vi "Test_Observe_NoPublication_Timeout.vi"(8 "error in (no error)":errorcluster, 11 "TestObservation In":refnum<class "TestPubSubRouting.lvclass">) -> (0 "error out":errorcluster, 3 "TestObservation Out":refnum<class "TestPubSubRouting.lvclass">)   [LabVIEW 2017, in "TestPubSubRouting.lvlib" / "TestPubSubRouting.lvclass"]
uses:
  TestPubSubRouting.lvclass
  gpm_packages/@cs/mva-core/Source/Mediator/Mediator/Mediator.lvclass
  <vilib>/ActorFramework/Actor/Actor.lvclass
  ObservingViewable/ObservingViewable.lvclass
  <vilib>/ActorFramework/Stop Msg/Stop Msg.lvclass
  ObservingViewModel/ObservingViewModel.lvclass
  ObservingModel/ObservingModel.lvclass
  41be6b66-6851-409e-b7f3-4ca1eaa927d9.vi
  C:/Program Files (x86)/National Instruments/LabVIEW 2017/vi.lib/ActorFramework/Actor/Actor.lvclass
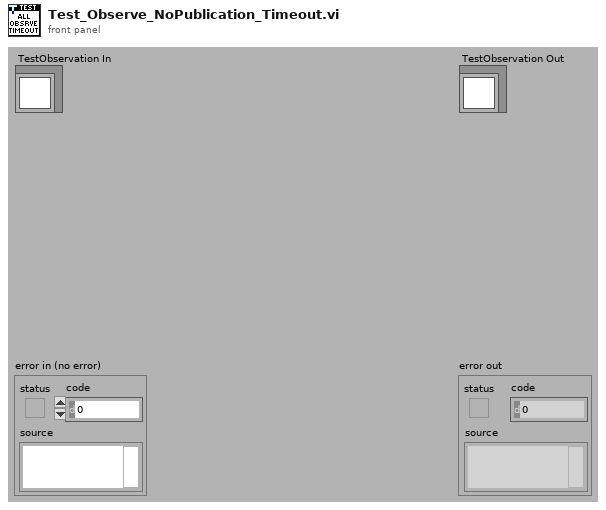
[diagram p1: front panel]
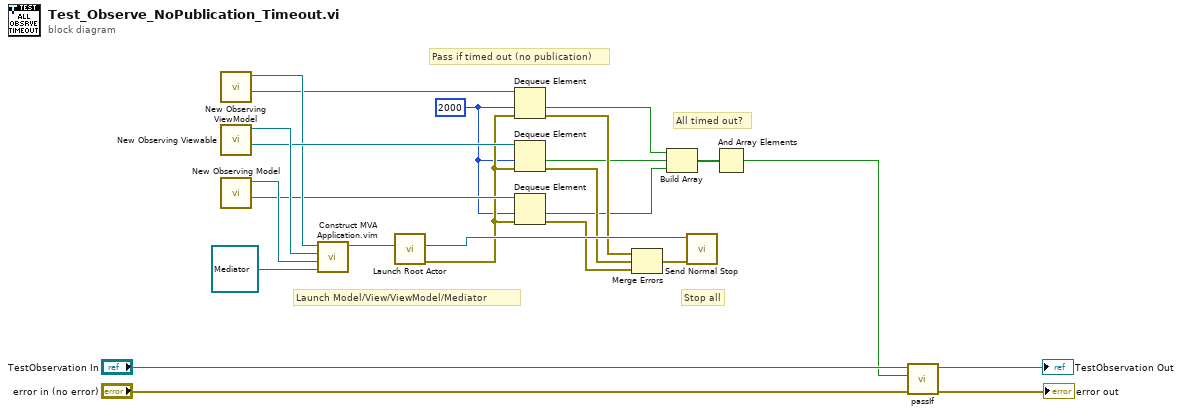
[diagram p0: block diagram]
diagram:
  w10 = 2000 ("timeout in ms (-1)")
  # "All timed out?"
  # "Stop all"
  # "Launch Model/View/ViewModel/Mediator"
  # "Pass if timed out (no publication)"
  n1 = call "New Observing ViewModel.vi"() -> ("Test Reply Queue"=w13:refnum<queue>, "ObservingViewModel Out"=w15:refnum<class "ObservingViewModel.lvclass">)  [unwired: 10 in]
  n2 = call "New Observing Viewable.vi"() -> ("Test Reply Queue"=w17:refnum<queue>, "ObservingViewable out"=w18:refnum<class "ObservingViewable.lvclass">)  [unwired: 10 in]
  n3 = call "New Observing Model.vi"() -> ("Test Reply Queue"=w12:refnum<queue>, "ObservingModel Out"=w14:refnum<class "ObservingModel.lvclass">)  [unwired: 10 in]
  n4 = call "Construct MVA Application.vim"("Mediator Type"=refnum<class "Mediator.lvclass"> refnum ("Mediator.lvlib:Mediator.lvclass"), "Model Type"=w14, "Startup View Configuration"=w18, "IViewModel In"=w15) -> ("IViewModel Out"=w19:refnum<class "ObservingViewModel.lvclass">)  [unwired: 7 in]
  n5 = call <vilib>:"Launch Root Actor.vi"("Actor"=w19) -> ("error out"=w11:errorcluster, "Actor's Enqueuer"=w16:refnum<class "Message Enqueuer.lvclass">)  [unwired: 9 in]
  n6 = Dequeue Element(queue=w13, timeout in ms (-1)=w10, error in (no error)=w11) -> (timed out?=w4:bool, error out=w9:errorcluster)  [unwired: 2 out]
  n7 = Dequeue Element(queue=w17, timeout in ms (-1)=w10, error in (no error)=w11) -> (timed out?=w3:bool, error out=w8:errorcluster)  [unwired: 2 out]
  n8 = Dequeue Element(queue=w12, timeout in ms (-1)=w10, error in (no error)=w11) -> (timed out?=w2:bool, error out=w7:errorcluster)  [unwired: 2 out]
  n9 = Merge Errors(w9, w8, w7) -> (w6:errorcluster)
  n10 = Build Array(w4, w3, w2) -> (w5:bool[])
  n11 = call <vilib>:"Send Normal Stop.vi"("error in (no error)"=w6, "Message Enqueuer"=w16) -> ()  [unwired: 9 in, 1 out]
  n12 = And Array Elements(Boolean array=w5) -> (logical AND=w1:bool)
  n13 = call-dynamic "passIf.vi"("error in (no error)"="error in (no error)", "pass"=w1, "TestCase in"="TestObservation In") -> ("error out"=→"error out":errorcluster, "TestCase out"=→"TestObservation Out":refnum<class "TestPubSubRouting.lvclass">)  [unwired: 7 in]
